vi "Reset_Instr.vi"(8 "error in (no error)":errorcluster caption="entrée d'erreur (pas d'erreur)", 11 "Class DIO en entrée":refnum<class "Class Instrument Ana.lvclass">) -> (0 "error out":errorcluster caption="sortie d'erreur", 3 "Class DIO en Sortie":refnum<class "Class Instrument Ana.lvclass">)   [LabVIEW 2020, in "Library Instrument & Equipement.lvlib" / "Library Instruments.lvlib" / "Class Instrument Ana.lvclass"]
uses:
  Class Instrument Ana.lvclass
  Class Instrument Ana.lvclass/Class Instrument Ana.ctl
  Instrument (Default)/Class Instrument (Default).lvclass
  Ana/Class Ana (Default)/Class Ana (Default).lvclass
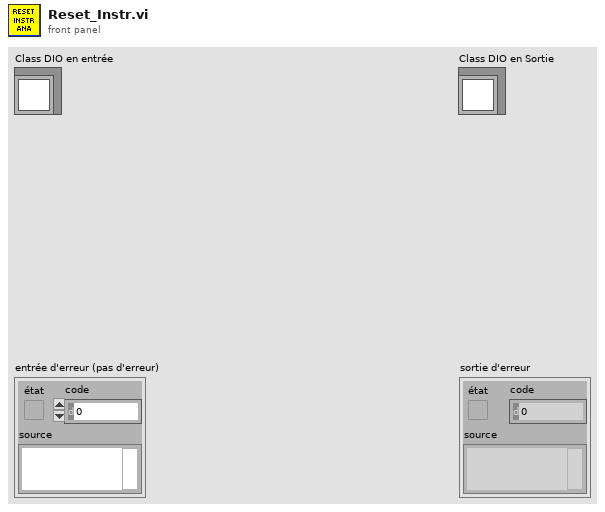
[diagram p1: front panel]
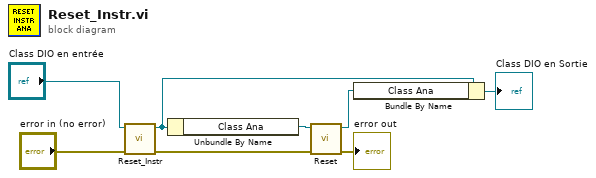
[diagram p0: block diagram]
diagram:
  n1 = call-parent "Reset_Instr.vi"("error in (no error)"="error in (no error)", "Class Instrument (Default) en entrée"="Class DIO en entrée") -> ("error out"=w4:errorcluster, "Class Instrument (Default) en sortie"=w5:refnum<class "Class Instrument Ana.lvclass">)  [unwired: 8 in]
  n2 = Unbundle By Name(w5) -> ("Class Ana"=w2:refnum<class "Class Ana (Default).lvclass">)
  n3 = call-dynamic "Reset.vi"("error in (no error)"=w4, "Class DIO (Default) en entrée"=w2) -> ("error out"=→"error out":errorcluster, "Class DIO (Default) en sortie"=w1:refnum<class "Class Ana (Default).lvclass">)  [unwired: 8 in]
  n4 = Bundle By Name(cluster=w5, "Class Ana"=w1) -> (→"Class DIO en Sortie":refnum<class "Class Instrument Ana.lvclass">)
